vi "Print Error.vi"(8 "Error In":errorcluster, 11 "Custom Device Name":string) -> ()   [LabVIEW 2020, in "Ballard MIL-STD-1553 Engine.lvlib" / "Custom Device.lvlib"]
doc: "Print detailed error information to VeriStand concole and log."
uses:
  Custom Device.lvlib
  <vilib>/Utility/error.llb/DialogType.ctl
  <vilib>/NI VeriStand/Custom Device Tools/Custom Device Utility Library/Custom Device Utility Library.lvlib
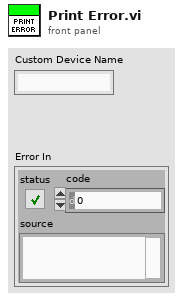
[diagram p1: front panel]
types:
  T1 = typedef "DialogType.ctl" = u16
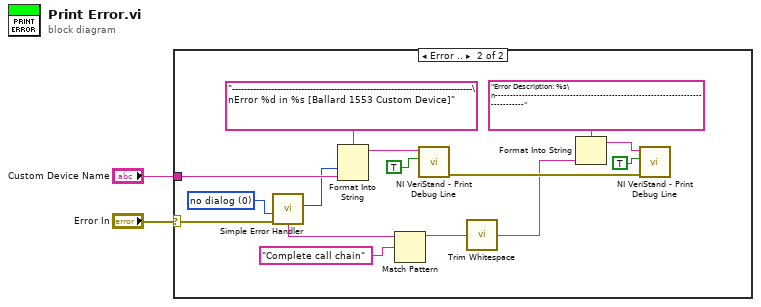
[diagram p0: block diagram]
diagram:
  n1 = case shown="Error .." "Error In" {
    selector: "Error In" -> [_ w9]
    tunnel: "Custom Device Name" -> [_ w16]
    frame No Error {
    }
    frame Error {
      w7 = T1 0 items=["no dialog", "OK message", "continue or stop message", "OK message + warnings", "continue/stop + warnings"] ("type of dialog (OK msg:1)")
      n2 = call <vilib>:"Simple Error Handler.vi"("type of dialog (OK msg:1)"=w7, "error in (no error)"=w9) -> ("code out"=w8:i32, "message"=w5:string)  [unwired: 3 in, 3 out]
      n3 = Format Into String(format string="--------------------------------------------------------------------------------\nError %d in %s [Ballard 1553 Custom Device]", w8, w16) -> (resulting string=w15:string)  [unwired: 2 in, 1 out]
      n4 = Match Pattern(string=w5, regular expression="Complete call chain") -> (before substring=w4:string)  [unwired: 1 in, 3 out]
      n5 = call <vilib>:"NI VeriStand - Print Debug Line.vi"("Add to log file? (F)"=TRUE, "Message"=w15) -> ("error out"=w11:errorcluster)  [unwired: 9 in]
      n6 = call <vilib>:"Trim Whitespace.vi"("string"=w4) -> ("trimmed string"=w3:string)  [unwired: 1 in]
      n7 = Format Into String(format string="Error Description: %s\n--------------------------------------------------------------------------------", w3) -> (resulting string=w12:string)  [unwired: 2 in, 1 out]
      n8 = call <vilib>:"NI VeriStand - Print Debug Line.vi"("error in (no error)"=w11, "Add to log file? (F)"=TRUE, "Message"=w12) -> ()  [unwired: 8 in, 1 out]
    }
  }
